vi "Quarternion SLERP.vi"(8 "error in (no error)":errorcluster, 9 "Factor":dbl, 10 "To":T1, 11 "From":T1) -> (0 "error out":errorcluster, 3 "SLERP Result":T1)   [LabVIEW 2020, in "g_ar_toolkit.ar.lvlib"]
uses:
  g_ar_toolkit.ar.lvlib
  Quaternion.ctl
  g_ar_toolkit.common/g_ar_toolkit.common.lvlib
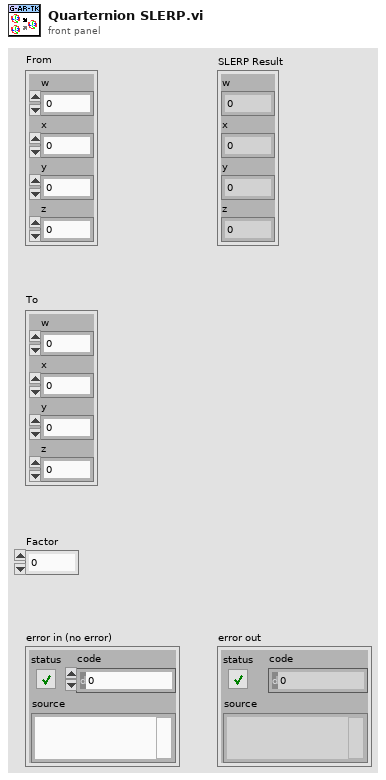
[diagram p1: front panel]
types:
  T1 = typedef "g_ar_toolkit.ar.lvlib/Quaternion.ctl" = cluster{"w":dbl, "x":dbl, "y":dbl, "z":dbl}
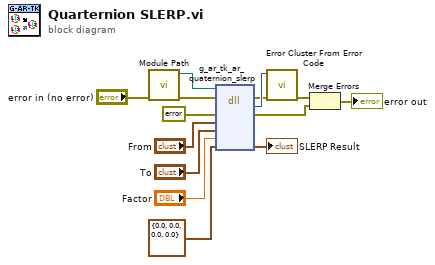
[diagram p0: block diagram]
diagram:
  n1 = call "Module Path.vi"("error in (no error)"="error in (no error)") -> ("error out"=w7:errorcluster, "Path"=w6:path)  [unwired: 9 in]
  n2 = dll-call lib="?" fn="g_ar_tk_ar_quaternion_slerp" ("g_ar_toolkit.*.*:g_ar_tk_image_copy")(path in=w6, error in=w7, "error_cluster"=errorcluster {"status"=FALSE, "code"=0, "source"=""} ("error constant"), "from"="From", "to"="To", "factor"="Factor", "result"=T1 {"w"=0.0, "x"=0.0, "y"=0.0, "z"=0.0} ("Quaternion")) -> (error out=w9:errorcluster, "MgErr"=w10:i32, "error_cluster"=w13:errorcluster, "result"=→"SLERP Result":T1)  [unwired: 4 in, 1 out]
  n3 = call <vilib>:"Error Cluster From Error Code.vi"("error in (no error)"=w9, "error code (0)"=w10) -> ("error out"=w11:errorcluster)  [unwired: 7 in]
  n4 = Merge Errors(w11, w13) -> (→"error out":errorcluster)
